vi "SmartSEM Remote API FIB probe currents.vi"(8 "error in":errorcluster, 10 "FIB Probe":string(combo), 11 "ActiveX Container":refnum<k7>(container)) -> (0 "error out":errorcluster, 1 "FIB probe current array":sgl[](array[numeric]), 2 "FIB probe array":string[](array[string]), 3 "reference out":refnum<k7>, 4 "Min probe current (nA)":sgl, 5 "Max probe current (nA)":sgl, 6 "Min probe":string, 7 "Max probe":string)   [LabVIEW 2018]
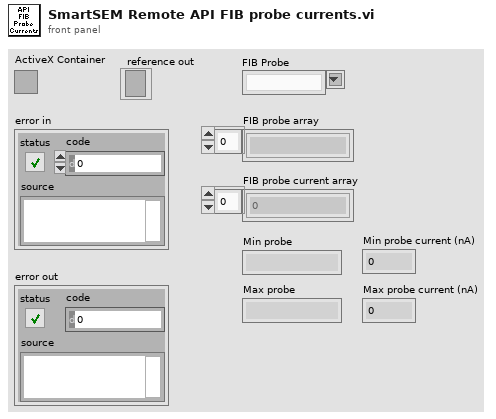
[diagram p1: front panel]
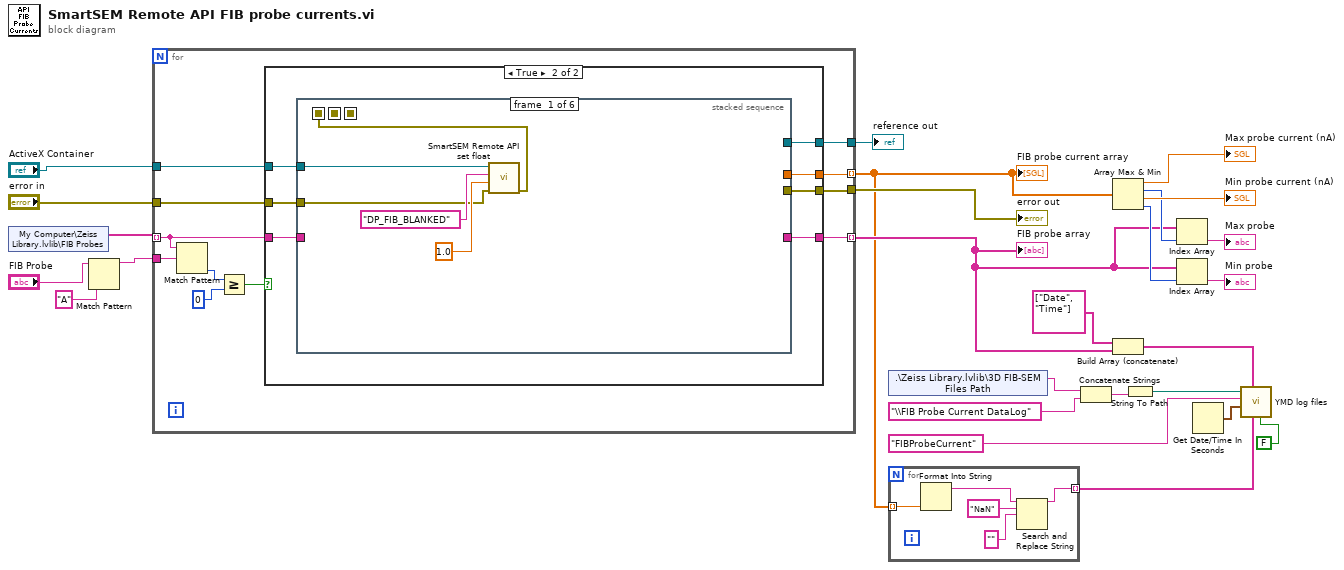
[diagram p0: block diagram]
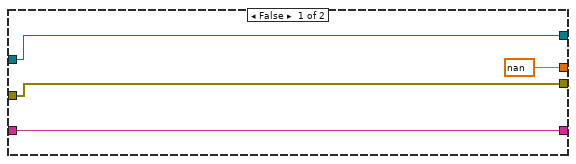
[diagram p2: hidden frame]
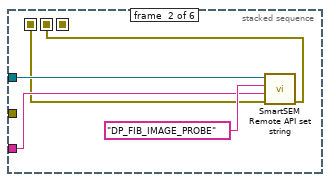
[diagram p3: hidden frame]
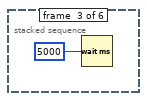
[diagram p4: hidden frame]
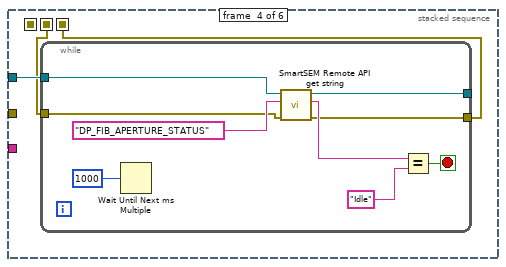
[diagram p5: hidden frame]
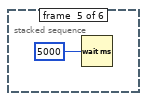
[diagram p6: hidden frame]
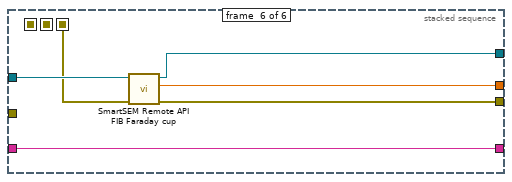
[diagram p7: hidden frame]
diagram:
  n1 = shared-variable "My Computer\\Zeiss Library.lvlib\\FIB Probes"() -> (w7:string[])  [unwired: 1 in, 1 out]
  n2 = Match Pattern(string="FIB Probe", regular expression="A") -> (before substring=w5:string)  [unwired: 1 in, 3 out]
  n3 = for {
    tunnel: "ActiveX Container" -> [w37]
    tunnel: [w36] -> w3 mode=indexing
    tunnel: [w35] -> w26
    tunnel: [w34] -> w25
    tunnel: [w33] -> w15 mode=indexing
    tunnel: w7 -> [w28] mode=indexing
    tunnel: w5 -> [w30]
    tunnel: "error in" -> [w27]
    n4 = Match Pattern(string=w28, regular expression=w30) -> (offset past match=w31:i32)  [unwired: 1 in, 3 out]
    n5 = Greater Or Equal?(x=w31, y=0) -> (x >= y?=w29:bool)
    n6 = case shown="True" w29 {
      tunnel: w37 -> [w40 w48]
      tunnel: [sgl nan ("FIB Faraday Cup (nA)") w47] -> w36
      tunnel: [w40 w46] -> w35
      tunnel: [w38 w45] -> w34
      tunnel: [w41 w44] -> w33
      tunnel: w28 -> [w41 w43]
      tunnel: w27 -> [w38 w42]
      frame False {
      }
      frame True {
        n7 = stacked-sequence {
          seq-local: [w49 _ _ _ _ _] -> [_ w55 _ _ _ _]
          seq-local: [_ w54 _ _ _ _] -> [_ _ _ w61 _ _]
          seq-local: [_ _ _ w60 _ _] -> [_ _ _ _ _ w73]
          tunnel: w43 -> [_ w57 _ _ _ w76]
          tunnel: w48 -> [w53 w56 _ w62 _ w78]
          tunnel: [_ _ _ _ _ w77] -> w47
          tunnel: [_ _ _ _ _ w75] -> w46
          tunnel: [_ _ _ _ _ w74] -> w45
          tunnel: [_ _ _ _ _ w76] -> w44
          tunnel: w42 -> [w50 _ _ _ _ _]
          frame #0 {
            n8 = call "SmartSEM Remote API set float.vi"("error in"=w50, "vValue"=sgl 1.0, "lpszParam"="DP_FIB_BLANKED", "ActiveX Container"=w53) -> ("error out"=w49:errorcluster)  [unwired: 6 in, 1 out]
          }
          frame #1 {
            n9 = call "SmartSEM Remote API set string.vi"("error in"=w55, "vValue"=w57, "lpszParam"="DP_FIB_IMAGE_PROBE", "ActiveX Container"=w56) -> ("error out"=w54:errorcluster)  [unwired: 6 in, 1 out]
          }
          frame #2 {
            n10 = Wait (ms)(milliseconds to wait=u32 5000) -> ()  [unwired: 1 out]
          }
          frame #3 {
            n11 = while {
              tunnel: w62 -> [w68]
              tunnel: w61 -> [w65]
              tunnel: [w64] -> _
              tunnel: [w63] -> w60
              stop <- w69 stop-if-true
              n12 = Wait Until Next ms Multiple(millisecond multiple=u32 1000) -> ()  [unwired: 1 out]
              n13 = call "SmartSEM Remote API get string.vi"("error in"=w65, "lpszParam"="DP_FIB_APERTURE_STATUS", "ActiveX Container"=w68) -> ("error out"=w63:errorcluster, "data"=w66:string, "reference out"=w64:refnum<k7>)  [unwired: 6 in]
              n14 = Equal?(x=w66, y="Idle" ("lpszParam")) -> (x = y?=w69:bool)
            }
          }
          frame #4 {
            n15 = Wait (ms)(milliseconds to wait=u32 5000) -> ()  [unwired: 1 out]
          }
          frame #5 {
            n16 = call "SmartSEM Remote API FIB Faraday cup.vi"("error in"=w73, "ActiveX Container"=w78) -> ("error out"=w74:errorcluster, "FIB Faraday Cup (nA)"=w77:sgl, "reference out"=w75:refnum<k7>)  [unwired: 7 in]
          }
        }
      }
    }
  }
  "error out" <- w25
  "FIB probe current array" <- w3
  "FIB probe array" <- w15
  "reference out" <- w26
  n17 = shared-variable ".\\Zeiss Library.lvlib\\3D FIB-SEM Files Path"() -> (w11:string)  [unwired: 1 in, 1 out]
  n18 = for {
    tunnel: [w79] -> w12 mode=indexing
    tunnel: w3 -> [w83] mode=indexing
    n19 = Format Into String(w83) -> (resulting string=w80:string)  [unwired: 3 in, 1 out]
    n20 = Search and Replace String(input string=w80, search string="NaN", replace string="" ("replace string (\"\")")) -> (result string=w79:string)  [unwired: 5 in, 3 out]
  }
  n21 = Concatenate Strings(w11, "\\FIB Probe Current DataLog" ("Log file name")) -> (w9:string)
  n22 = Array Max & Min(array=w3) -> (max value=→"Max probe current (nA)":sgl, max index (indices)=w20:i32, min value=→"Min probe current (nA)":sgl, min index (indices)=w24:i32)
  n23 = Build Array (concatenate)(string[] ["Date", "Time"], w15) -> (w13:string[])
  n24 = String To Path(string=w9) -> (path=w8:path)
  n25 = Index Array(array=w15, index=w20) -> (element=→"Max probe":string)
  n26 = Index Array(array=w15, index=w24) -> (element=→"Min probe":string)
  n27 = Get Date/Time In Seconds() -> (seconds since 1Jan1904=w16:timestamp)
  n28 = call "YMD log files.vi"("Day"=FALSE ("Month"), "Input text array"=w12, "Input header array"=w13, "current time"=w16, "Log file name"="FIBProbeCurrent", "Log file path"=w8) -> ()  [unwired: 6 in]
